vi "MHM Load Register Ex.vi"(8 "error in (no error)":errorcluster, 9 "ulArraySize":u32=256, 10 "pcFilename":string, 11 "ulMHMHandle":u32) -> (0 "error out (no error)":errorcluster, 1 "pulValid":u32[](array[numeric]), 2 "pulData":u32[](array[numeric]), 3 "function return":u32)   [LabVIEW 2017, in "MHM_1SL_interface.lvlib"]
uses:
  MHM_1SL_interface.lvlib
  SSI_Tool/DUT_Interface/lv_interface/lib/MHM_1SL_interface.dll
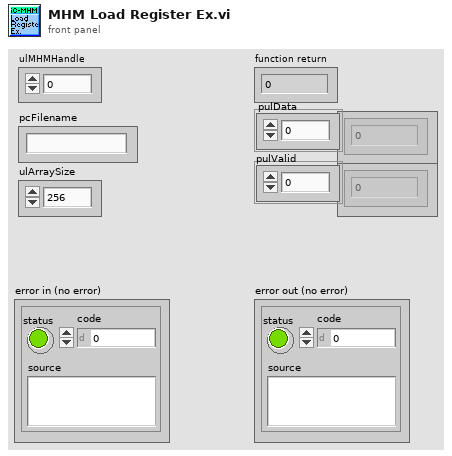
[diagram p1: front panel]
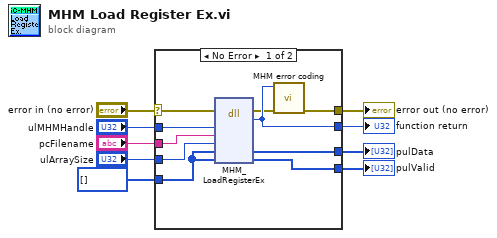
[diagram p0: block diagram]
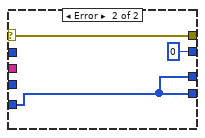
[diagram p2: hidden frame]
diagram:
  n1 = case shown="No Error" "error in (no error)" {
    selector: "error in (no error)" -> [w15 w22]
    tunnel: [w19 u32 0 ("return type")] -> w9
    tunnel: "ulMHMHandle" -> [w18 _]
    tunnel: [w16 w22] -> w7
    tunnel: "pcFilename" -> [w14 _]
    tunnel: "ulArraySize" -> [w13 _]
    tunnel: [w12 w20] -> w3
    tunnel: [w11 w20] -> w2
    tunnel: u32[] [] ("pulValid") -> [w10 w20]
    frame No Error {
      n2 = dll-call lib="C:/workspace/project/scancon/sw/SSI_Tool/DUT_Interface/lv_interface/lib/MHM_1SL_interface.dll" fn="MHM_LoadRegisterEx"(error in=w15, "ulMHMHandle"=w18, "pcFilename"=w14, "ulArraySize"=w13, "pulData"=w10, "pulValid"=w10) -> (error out=w17:errorcluster, "return type"=w19:u32, "pulData"=w12:u32[], "pulValid"=w11:u32[])  [unwired: 5 in, 1 out]
      n3 = call "MHM error coding.vi"("error in (no error)"=w17, "function return in"=w19) -> ("error out"=w16:errorcluster)  [unwired: 9 in]
    }
    frame Error {
    }
  }
  "function return" <- w9
  "error out (no error)" <- w7
  "pulData" <- w3
  "pulValid" <- w2
